vi "StepRange.vi"(9 "Step size (um)":dbl, 11 "Number of Steps":i32) -> (1 "Center Index":i32, 3 "Displacements (um)":dbl[](array[numeric]))   [LabVIEW 2015]
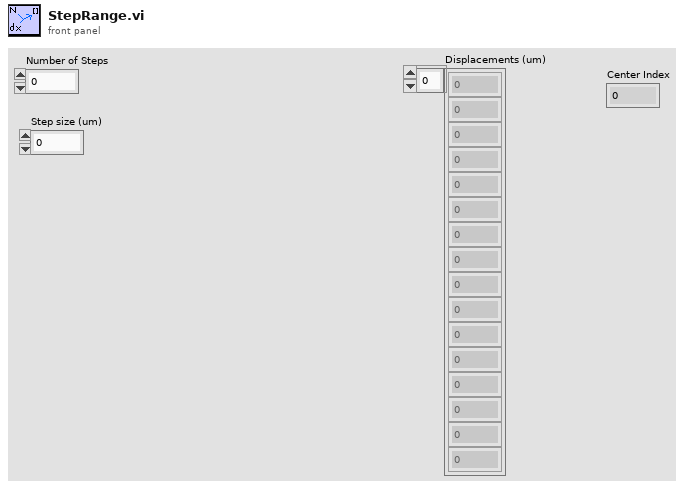
[diagram p1: front panel]
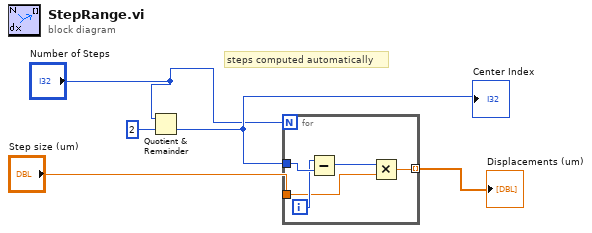
[diagram p0: block diagram]
diagram:
  # "steps computed automatically"
  n1 = Quotient & Remainder(x="Number of Steps", y=2) -> (floor(x/y)=w4:i32)  [unwired: 1 out]
  "Center Index" <- w4
  n2 = for {
    N: "Number of Steps" -> [_]
    tunnel: w4 -> [w10]
    tunnel: [w6] -> w1 mode=indexing
    tunnel: "Step size (um)" -> [w7]
    i -> [w9]
    n3 = Subtract(x=w9, y=w10) -> (x-y=w8:i32)
    n4 = Multiply(x=w8, y=w7) -> (x*y=w6:dbl)
  }
  "Displacements (um)" <- w1
